vi "BuildTestFromProjectItem_LibraryWithFact_BuildsTestSuiteWithFact.vi"() -> ()   [LabVIEW 2019, in "LVUnitTestBuilderTest.lvlib"]
uses:
  LVUnitTestBuilderTest.lvlib
  LVUnitTestBuilder/LVUnitTestBuilder.lvclass
  TestSuite/TestSuite.lvclass
  Fact/Fact.lvclass
  TestSuite/TestSuite.lvclass/TestSuite.ctl
  TestSuite/ReadTests.vi
  Test/Test.lvclass
  Assertion/Assertion.lvlib
panel:
  out "error out":errorcluster
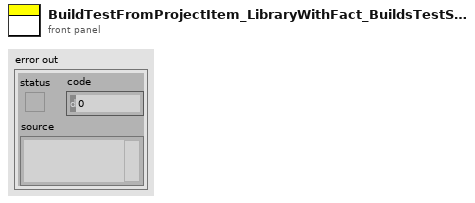
[diagram p1: front panel]
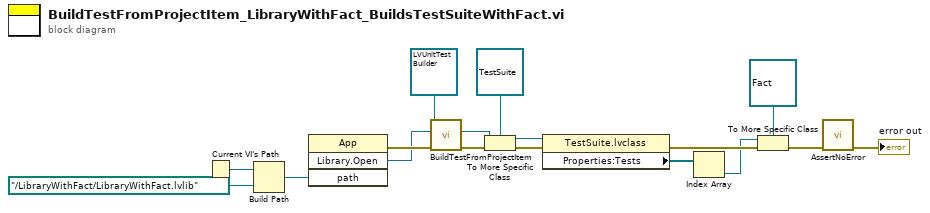
[diagram p0: block diagram]
diagram:
  n1 = Current VI's Path() -> (path=w10:path)
  n2 = Build Path(base path=w10, name or relative path=path "../LibraryWithFact/LibraryWithFact.lvlib") -> (appended path=w9:path)
  n3 = invoke class="App" method="Library.Open"("path"=w9) -> (error out=w13:errorcluster, "Open Library"=w12:refnum<vi>)  [unwired: 3 in, 2 out]
  n4 = call-dynamic "BuildTestFromProjectItem.vi"("error in (no error)"=w13, "ProjectItem Refnum"=w12, "LVUnitTestBuilder in"=refnum<class "LVUnitTestBuilder.lvclass"> refnum ("LVUnitTestBuilder")) -> ("error out"=w14:errorcluster, "Test"=w16:refnum<class "Test.lvclass">)  [unwired: 6 in, 1 out]
  n5 = To More Specific Class(target class=refnum<class "TestSuite.lvclass"> refnum ("TestSuite.lvclass"), reference=w16, error in=w14) -> (specific class reference=w7:refnum<class "TestSuite.lvclass">, error out=w8:errorcluster)
  n6 = property class="TestSuite.lvclass"(reference=w7, error in=w8) -> (error out=w5:errorcluster, "Properties:Tests"=w6:refnum<class "Test.lvclass">[])  [unwired: 1 out]
  n7 = Index Array(array=w6) -> (element=w3:refnum<class "Test.lvclass">)  [unwired: 1 in]
  n8 = To More Specific Class(target class=refnum<class "Fact.lvclass"> refnum ("TestCase.lvlib:Fact.lvclass"), reference=w3, error in=w5) -> (error out=w4:errorcluster)  [unwired: 1 out]
  n9 = call "AssertNoError.vi"("error in (no error)"=w4) -> ("error out"=→"error out":errorcluster)  [unwired: 10 in]
